vi "Copy.vi"(8 "error in (no error)":errorcluster {"code" format="%.0x"}, 9 "SourceTraceLimitIndex":i32=1 format="%.0g", 10 "DigitalDemodTraceLimit":string="TraceLimit1", 11 "instrument handle":refnum<k15>) -> (0 "error out":errorcluster {"code" format="%.0x"}, 3 "instrument handle out":refnum<k15>)   [LabVIEW 2021, in "Keysight XSAnVMA.lvlib"]
doc: "Copies an existing limit into the current limit, including all secondary parameters (Description, Comment, Associated Window, X Axis Unit, Y Axis Unit, X Offset, Y Offset, Type, Margin, X Reference)."
uses:
  <instrlib>/Keysight XSAnVMA/Keysight XSAnVMA.lvlib
  KtXSAnVMA_64.dll
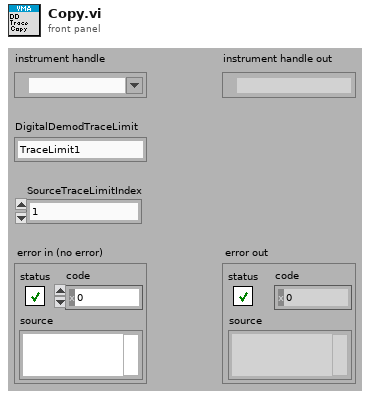
[diagram p1: front panel]
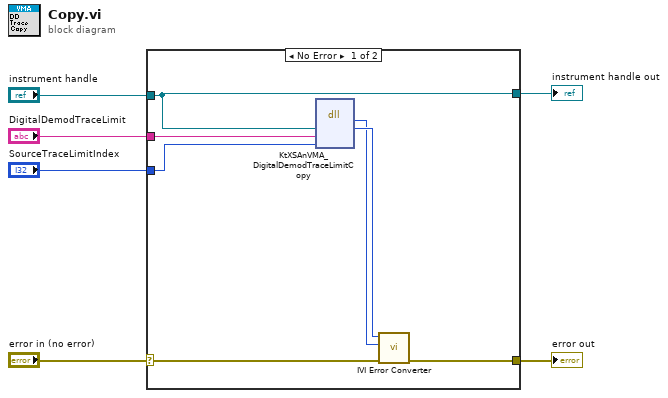
[diagram p0: block diagram]
diagram:
  n1 = case shown="No Error" "error in (no error)" {
    selector: "error in (no error)" -> [w11 w15]
    tunnel: [w10 w15] -> w6
    tunnel: "instrument handle" -> [w7 w14]
    tunnel: "DigitalDemodTraceLimit" -> [w9 _]
    tunnel: "SourceTraceLimitIndex" -> [w8 _]
    tunnel: [w7 w14] -> w1
    frame No Error {
      n2 = dll-call lib="KtXSAnVMA**.dll" fn="KtXSAnVMA_DigitalDemodTraceLimitCopy"("Vi"=w7, "DigitalDemodTraceLimit"=w9, "SourceTraceLimitIndex"=w8) -> (w12:i32, "Vi"=w13:u32)  [unwired: 5 in, 2 out]
      n3 = call <instrlib>:"IVI Error Converter.vi"("error in (no error)"=w11, "IVI error code (0)"=w12, "instrument handle"=w13) -> ("error out"=w10:errorcluster)  [unwired: 7 in, 1 out]
    }
    frame Error {
    }
  }
  "error out" <- w6
  "instrument handle out" <- w1
